vi "Get Linker Cache.vi"(7 "Status Ref":refnum<vi>, 8 "error in (no error)":errorcluster, 11 "WorkSpace / Repo path":path) -> (0 "error out":errorcluster, 1 "LV Version Mismatched VI":path[](array[path]), 2 "Status":string, 3 "Caller Map":map{string, string[]}(c390))   [LabVIEW 2019, in "Hawkeye.lvlib"]
uses:
  Hawkeye.lvlib
  f2e1f123-2e97-488a-9f38-c5ab8c69dbb8.vi
  3dc4041e-3bdf-4db9-bc93-15cebc6804b8.vi
  <userlib>/_OpenG.lib/array/array.llb/Search 1D Array (String)__ogtk.vi
panel:
  # "Generating Linker Cache file"
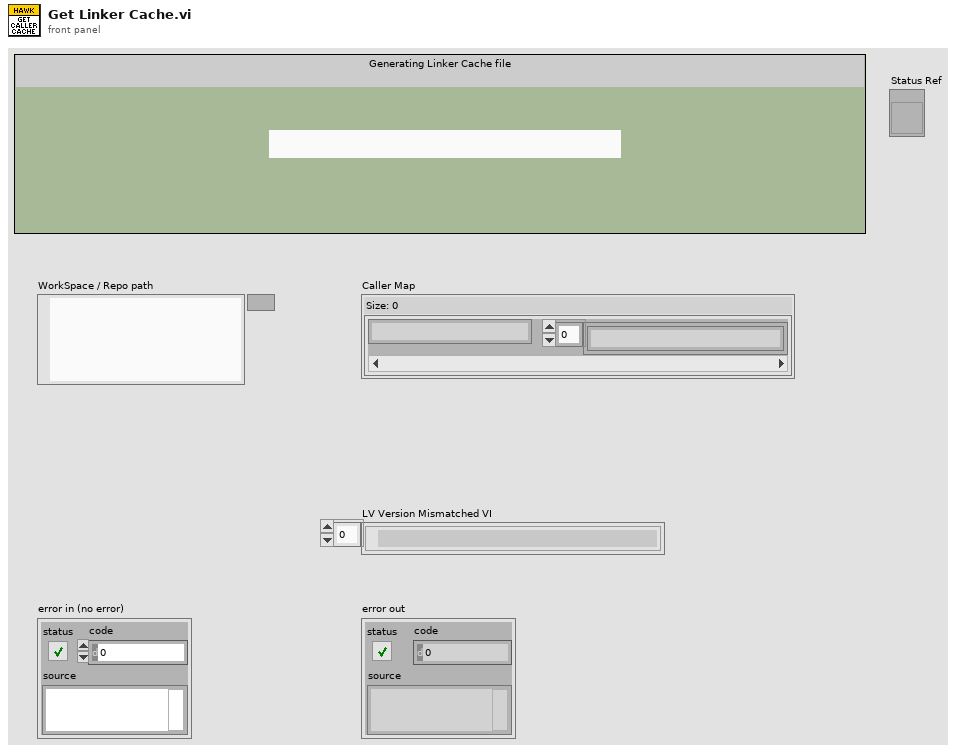
[diagram p1: front panel]
types:
  T1 = enum16{"open", "replace", "create", "open or create", "replace or create", "replace or create with confirmation"}
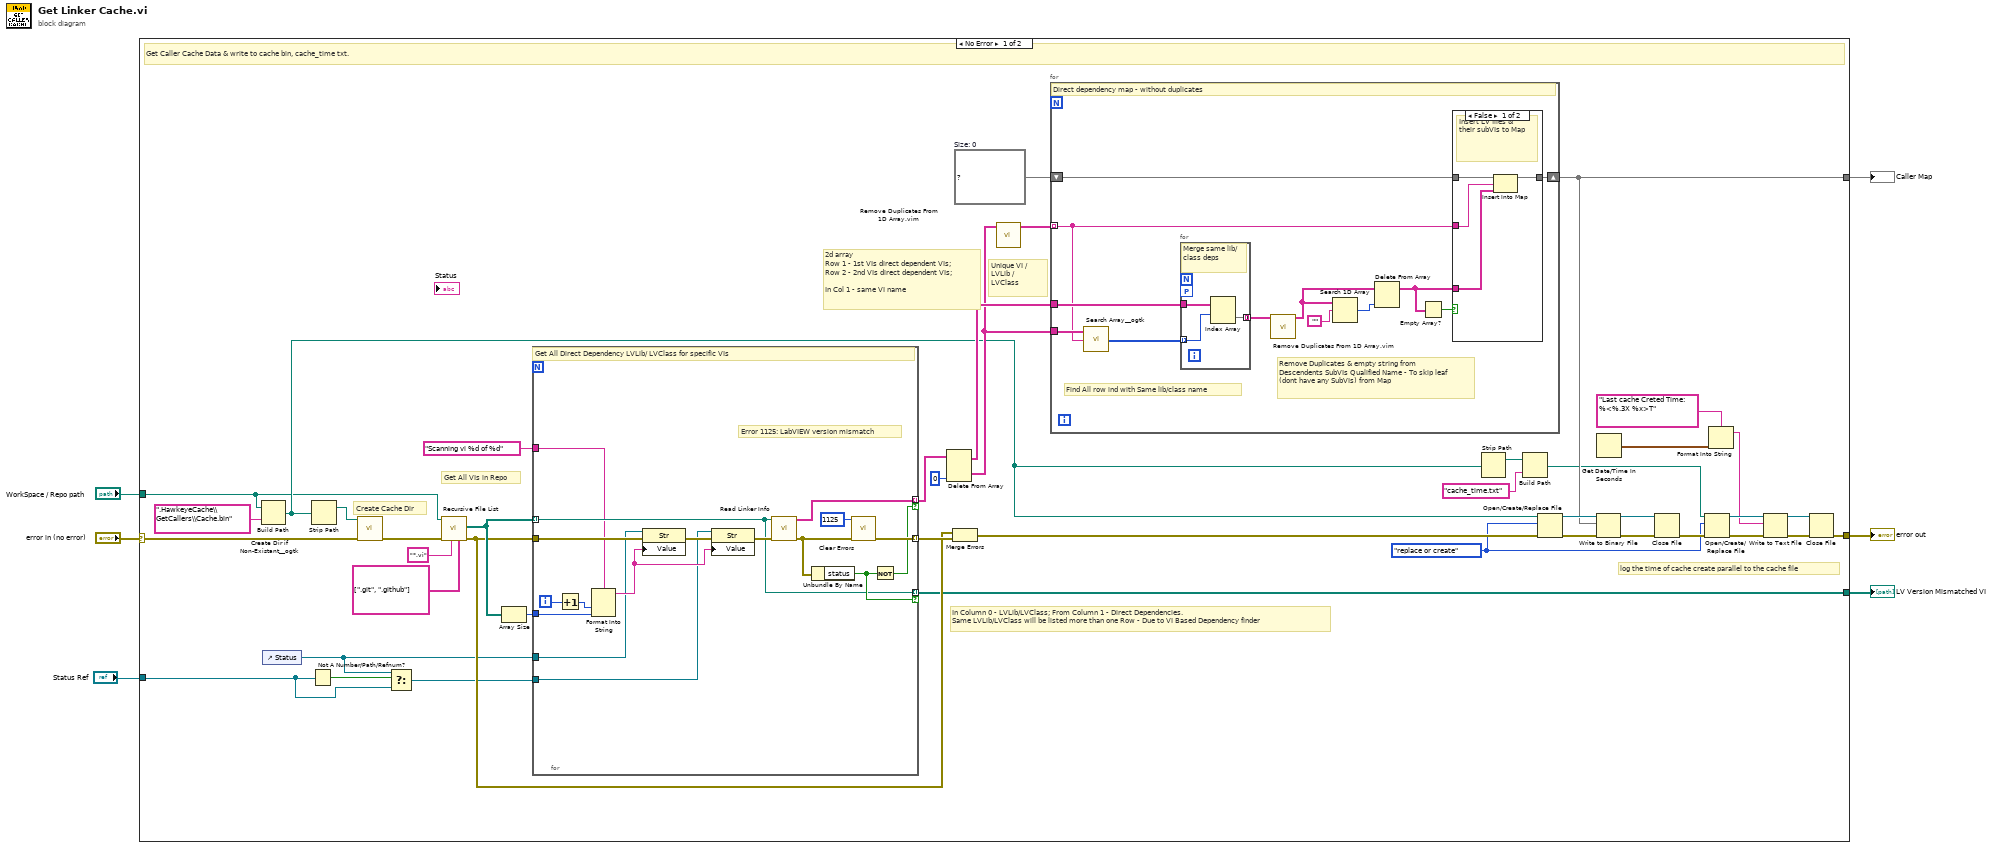
[diagram p0: block diagram]
diagram:
  n1 = case shown="No Error" "error in (no error)" {
    selector: "error in (no error)" -> [w47 w87]
    tunnel: [w32 _] -> w5
    tunnel: [w27 _] -> w4
    tunnel: [w17 w87] -> w3
    tunnel: "WorkSpace / Repo path" -> [w12 _]
    tunnel: "Status Ref" -> [w9 _]
    frame No Error {
      w16 = T1."replace or create" ("operation (0:open)")
      w33 = map{string, string[]} {}  # Size: 0
      # "Unique VI / LVLib / LVClass"
      # "log the time of cache create parallel to the cache file"
      # "2d array \nRow 1 - 1st VIs direct dependent VIs; \nRow 2 - 2nd VIs direct dependent VIs;\n\nIn Col 1 - same VI name"
      # "In Column 0 - LVLib/LVClass; From Column 1 - Direct Dependencies.\nSame LVLib/LVClass will be listed more than one Row - Due to VI Based Dependency finder"
      # "Get All VIs in Repo"
      # "Create Cache Dir"
      # "Get Caller Cache Data & write to cache bin, cache_time txt."
      n2 = Build Path(base path=w12, name or relative path=".HawkeyeCache\\GetCallers\\Cache.bin") -> (appended path=w20:path)
      n3 = control-ref of="Status"() -> (w8:refnum<vi>)
      n4 = Not A Number/Path/Refnum?(number/path/refnum=w9) -> (NaN/Path/Refnum?=w11:bool)
      n5 = Strip Path(path=w20) -> (stripped path=w48:path)  [unwired: 1 out]
      n6 = call <userlib>:"Create Dir if Non-Existant__ogtk.vi"("error in (no error)"=w47, "Directory Path"=w48) -> ("error out"=w46:errorcluster)  [unwired: 7 in, 2 out]
      n7 = Select(t=w8, s=w11, f=w9) -> (s? t:f=w10:refnum<vi>)
      n8 = call <vilib>:"Recursive File List.vi"("Folders to Exclude"=string[] [".git", ".github"], "pattern"="*.vi", "error in (no error)"=w46, "Folder Path"=w12) -> ("error out"=w29:errorcluster, "All Files in Dir"=w38:path[])  [unwired: 3 in, 3 out]
      n9 = Array Size(array=w38) -> (size(s)=w43:i32)
      n10 = for {
        tunnel: w43 -> [w86]
        tunnel: [w79] -> w36 mode=indexing if=w81
        tunnel: w29 -> [w75]
        tunnel: w38 -> [w71] mode=indexing
        tunnel: [w84] -> w31 mode=indexing
        tunnel: [w71] -> w27 mode=indexing if=w82
        tunnel: w10 -> [w73]
        tunnel: w8 -> [w72]
        tunnel: "Scanning vi %d of %d" ("format string") -> [w70]
        i -> [w80]
        # "Error 1125: LabVIEW version mismatch"
        # "Get All Direct Dependency LVLib/ LVClass for specific VIs"
        n11 = Increment(x=w80) -> (x+1=w85:i32)
        n12 = Format Into String(format string=w70, w85, w86) -> (resulting string=w74:string)  [unwired: 2 in, 1 out]
        n13 = property class="Str"(reference=w72, error in=w75, "Value"=w74) -> (error out=w77:errorcluster)  [unwired: 1 out]
        n14 = property class="Str"(reference=w73, error in=w77, "Value"=w74) -> (error out=w76:errorcluster)  [unwired: 1 out]
        n15 = call "Read Linker Info.vi"("error in (no error)"=w76, "VI Path"=w71) -> ("error out"=w78:errorcluster, "All VI Dependencies"=w79:string[])  [unwired: 8 in]
        n16 = Unbundle By Name(w78) -> ("status"=w82:bool)
        n17 = call <vilib>:"Clear Errors.vi"("error in (no error)"=w78, "specific error code to clear (0: all)"=1125) -> ("error out"=w84:errorcluster)  [unwired: 4 in, 1 out]
        n18 = Not(x=w82) -> (.not. x?=w81:bool)
      }
      n19 = Delete From Array(array=w36, index (col)=0 ("disabled index (col)")) -> (deleted portion=w34:string[], array with subset deleted=w35:string[][])  [unwired: 2 in]
      n20 = Merge Errors(w29, w31) -> (w30:errorcluster)
      n21 = call "Remove Duplicates From 1D Array.vim"("array"=w34) -> ("array with duplicates removed"=w28:string[])  [unwired: 10 in]
      n22 = for {
        tunnel: w28 -> [w57] mode=indexing
        tunnel: w34 -> [w61]
        shift-right: [w58] -> w32
        shift-left: w33 -> [w60]
        tunnel: w35 -> [w59]
        # "Find All row ind with Same lib/class name"
        # "Remove Duplicates & empty string from \nDescendents SubVIs Qualified Name - To skip leaf (dont have any SubVIs) from Map"
        # "Direct dependency map - without duplicates"
        n23 = call-poly <userlib>:"Search Array__ogtk.vi"("Array"=w61, "Element Data"=w57) -> ("Indices of Elements"=w51:i32[])  [unwired: 7 in]
        n24 = for {
          tunnel: w59 -> [w64]
          tunnel: w51 -> [w63] mode=indexing
          tunnel: [w62] -> w50 mode=concatenating
          workers-P: _ -> [_]
          # "Merge same lib/class deps"
          n25 = Index Array(array=w64, index (row)=w63) -> (element=w62:string[])  [unwired: 1 in]
        }
        n26 = call "Remove Duplicates From 1D Array.vim"("array"=w50) -> ("array with duplicates removed"=w54:string[])  [unwired: 10 in]
        n27 = Search 1D Array(1D array=w54, element="" ("Empty String Constant")) -> (index of element=w55:i32)  [unwired: 1 in]
        n28 = Delete From Array(array=w54, index=w55) -> (array with subset deleted=w52:string[])  [unwired: 1 in, 1 out]
        n29 = Empty Array?(array=w52) -> (empty?=w53:bool)
        n30 = case shown="False" w53 {
          tunnel: [w68 w69] -> w58
          tunnel: w60 -> [w67 w69]
          tunnel: w57 -> [w65 _]
          tunnel: w52 -> [w66 _]
          frame False {
            # "Insert LV files & their subVIs to Map"
            n31 = Insert Into Map(map in=w67, key=w65, value=w66) -> (map out=w68:map{string, string[]})  [unwired: 2 out]
          }
          frame True {
          }
        }
      }
      n32 = Strip Path(path=w20) -> (stripped path=w22:path)  [unwired: 1 out]
      n33 = Build Path(base path=w22, name or relative path="cache_time.txt") -> (appended path=w19:path)
      n34 = Open/Create/Replace File(file path (use dialog)=w20, error in=w30, operation (0:open)=w16) -> (refnum out=w42:refnum<file>, error out=w39:errorcluster)  [unwired: 3 in, 1 out]
      n35 = Write to Binary File(file (use dialog)=w42, data=w32, error in=w39) -> (refnum out=w41:refnum<file>, error out=w40:errorcluster)  [unwired: 3 in, 1 out]
      n36 = Get Date/Time In Seconds() -> (seconds since 1Jan1904=w14:timestamp)
      n37 = Close File(refnum=w41, error in=w40) -> (error out=w18:errorcluster)  [unwired: 1 out]
      n38 = Open/Create/Replace File(file path (use dialog)=w19, error in=w18, operation (0:open)=w16) -> (refnum out=w24:refnum<file>, error out=w26:errorcluster)  [unwired: 3 in, 1 out]
      n39 = Format Into String(format string="Last cache Creted Time: %<%.3X %x>T" ("name or relative path"), w14) -> (resulting string=w13:string)  [unwired: 2 in, 1 out]
      n40 = Write to Text File(file (use dialog)=w24, text=w13, error in=w26) -> (refnum out=w23:refnum<file>, error out=w25:errorcluster)  [unwired: 1 in, 1 out]
      n41 = Close File(refnum=w23, error in=w25) -> (error out=w17:errorcluster)  [unwired: 1 out]
    }
    frame Error {
    }
  }
  "error out" <- w3
  "Caller Map" <- w5
  "LV Version Mismatched VI" <- w4
